vi "DecodeFloat.vi"(1 "Data In":u8[](array[numeric])) -> (0 "Data Out":fxp<+/-,32,16>[](array[numeric]) format="%.4f")   [LabVIEW 2014, in "navX Library v1 (deprecated).lvlib"]
uses:
  navX Library v1 (deprecated).lvlib
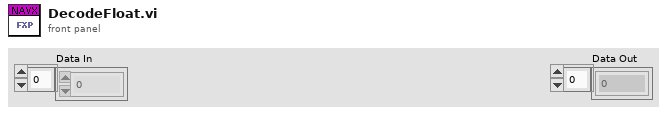
[diagram p1: front panel]
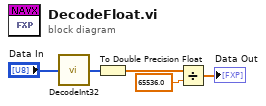
[diagram p0: block diagram]
diagram:
  n1 = call "DecodeInt32.vi"("Data In"="Data In") -> ("Data Out"=w4:i32[])
  n2 = To Double Precision Float(number=w4) -> (double precision float=w2:dbl[])
  n3 = Divide(x=w2, y=65536.0) -> (x/y=→"Data Out":dbl[])
